vi "Check_Connections_between_Displ_in_Tracks-1.vi"(4 "error IN":errorcluster, 7 "[IN] Long Connected Tracks":T1(array[cluster])) -> (0 "error OUT":errorcluster, 3 "[OUT] Long Connected Tracks":T1(array[cluster]))   [LabVIEW 2013]
panel:
  out "Number of Unconnected Points":u8
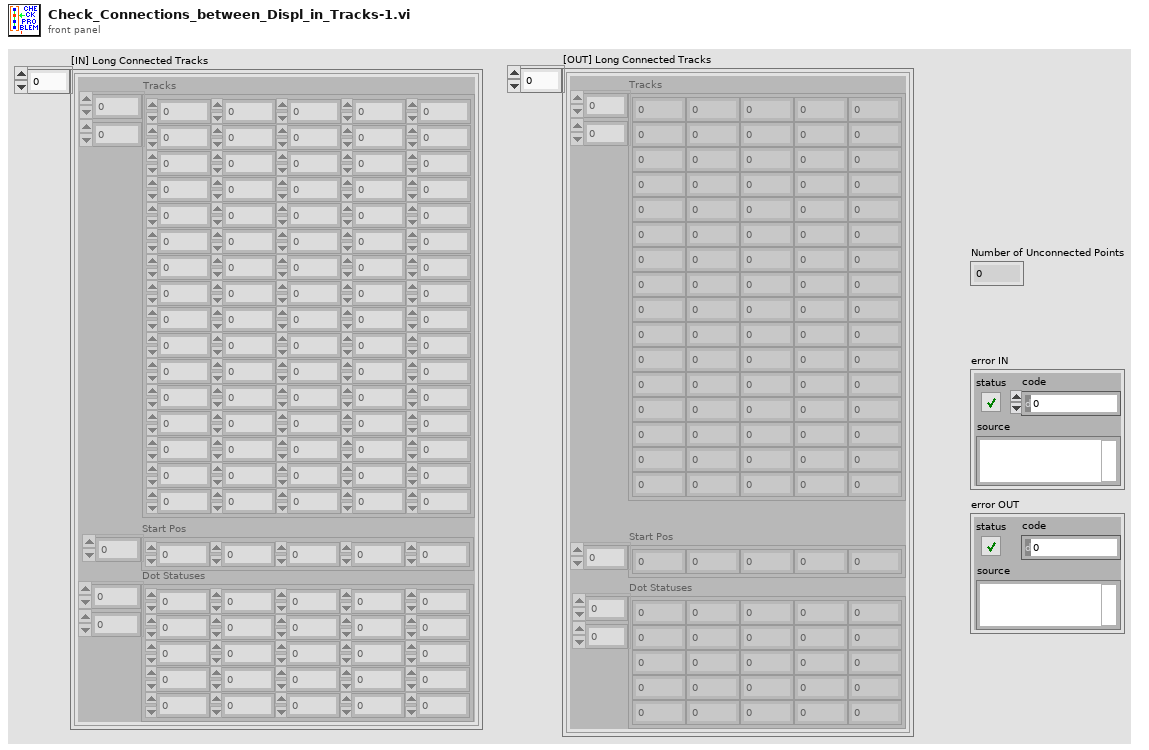
[diagram p1: front panel]
types:
  T1 = cluster{"Tracks":dbl[][], "Start Pos":i32[], "Dot Statuses":i16[][]}[]
  T2 = cluster{"Tracks":dbl[][], "Start Pos":i32[], "Dot Statuses":i16[][]}
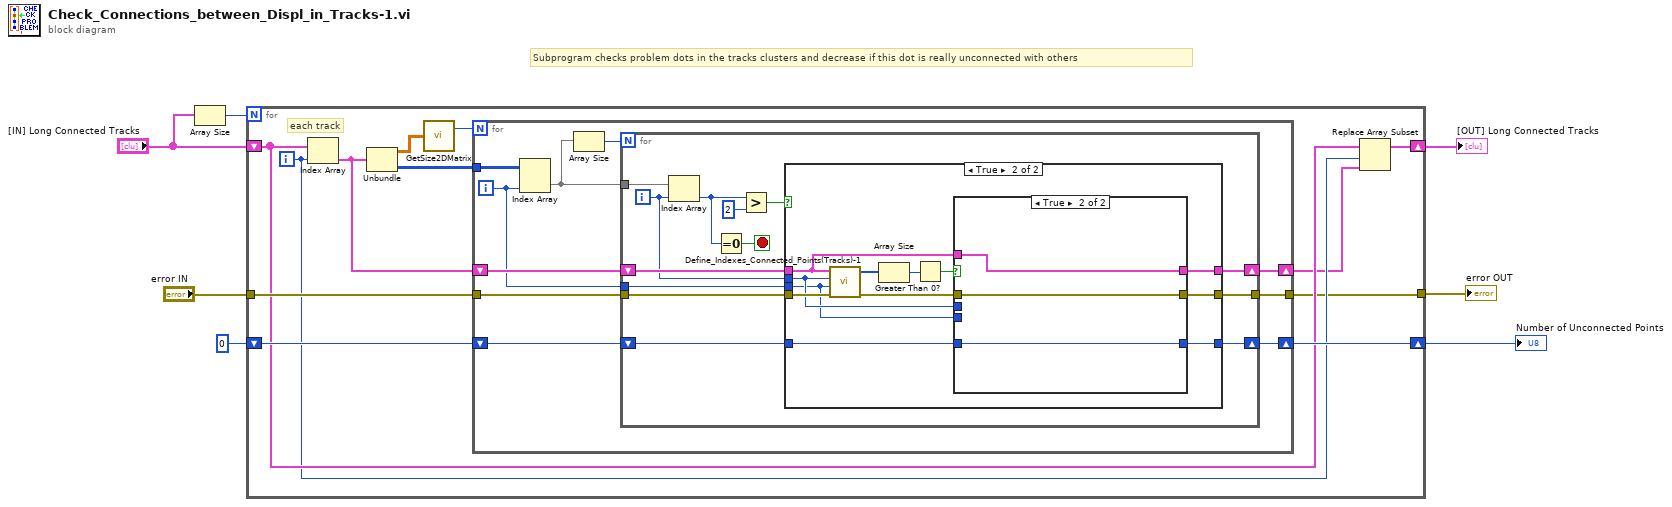
[diagram p0: block diagram]
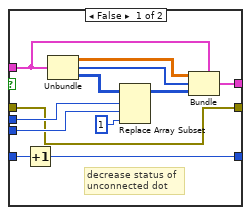
[diagram p3: hidden frame]
diagram:
  # "Subprogram checks problem dots in the tracks clusters and decrease if this dot is really unconnected with others"
  n1 = Array Size(array="[IN] Long Connected Tracks") -> (size(s)=w7:i32)
  n2 = for {
    N: w7 -> [_]
    shift-right: [w9] -> w2
    shift-left: "[IN] Long Connected Tracks" -> [w12]
    tunnel: "error IN" -> [w15]
    shift-right: [w13] -> w1
    shift-left: u8 0 -> [w14]
    tunnel: [w8] -> w3
    i -> [w11]
    # "each track"
    n3 = Index Array(array=w12, index=w11) -> (element=w16:T2)
    n4 = Unbundle(w16) -> ("Tracks"=w19:dbl[][], "Dot Statuses"=w17:i16[][])  [unwired: 1 out]
    n5 = call "GetSize2DMatrix.vi"("Array IN (2D)"=w19) -> ("# Cols"=w18:i32)  [unwired: 1 out]
    n6 = for {
      N: w18 -> [_]
      tunnel: w17 -> [w29]
      shift-right: [w23] -> w10
      shift-left: w16 -> [w26]
      tunnel: w15 -> [w24]
      shift-right: [w21] -> w13
      shift-left: w14 -> [w22]
      tunnel: [w20] -> w8
      i -> [w25]
      n7 = Index Array(array=w29, index (col)=w25) -> (element=w27:i16[])  [unwired: 1 in]
      n8 = Array Size(array=w27) -> (size(s)=w28:i32)
      n9 = for {
        N: w28 -> [_]
        tunnel: w27 -> [w42]
        shift-right: [w33] -> w23
        shift-left: w26 -> [w38]
        tunnel: w25 -> [w35]
        tunnel: w24 -> [w34]
        shift-right: [w31] -> w21
        shift-left: w22 -> [w32]
        tunnel: [w30] -> w20
        i -> [w36]
        stop <- w41 stop-if-true
        n10 = Index Array(array=w42, index=w36) -> (element=w37:i16)
        n11 = Equal To 0?(x=w37) -> (x = 0?=w41:bool)
        n12 = Greater?(x=w37, y=i16 2) -> (0:w39:bool)
        n13 = case shown="True" w39 {
          tunnel: w38 -> [w45 w53]
          tunnel: w36 -> [_ w49]
          tunnel: w35 -> [_ w48]
          tunnel: w34 -> [w44 w57]
          tunnel: [w45 w52] -> w33
          tunnel: w32 -> [w43 w51]
          tunnel: [w43 w50] -> w31
          tunnel: [w44 w46] -> w30
          frame False {
          }
          frame True {
            n14 = call "Define_Indexes_Connected_Points(Tracks)-1.vi"("error IN"=w57, "[IN] Index of track with\n(problem displacement)"=w48, "[IN]Index of problem\ndisplacement inside track"=w49, "[IN] Track group"=w53) -> ("error OUT"=w47:errorcluster, "[OUT] Index of connected\ntracks with problem dot"=w56:i32[])  [unwired: 1 out]
            n15 = Array Size(array=w56) -> (size(s)=w55:i32)
            n16 = Greater Than 0?(x=w55) -> (x > 0?=w54:bool)
            n17 = case shown="True" w54 {
              tunnel: w53 -> [w67 w72]
              tunnel: [w66 w72] -> w52
              tunnel: w51 -> [w69 w70]
              tunnel: [w68 w70] -> w50
              tunnel: w49 -> [w64 _]
              tunnel: w48 -> [w63 _]
              tunnel: w47 -> [w58 w71]
              tunnel: [w58 w71] -> w46
              frame False {
                # "decrease status of \nunconnected dot"
                n18 = Increment(x=w69) -> (x+1=w68:u8)
                n19 = Unbundle(w67) -> ("Tracks"=w62:dbl[][], "Start Pos"=w61:i32[], "Dot Statuses"=w65:i16[][])
                n20 = Replace Array Subset(array=w65, new element=i16 1 ("new element/subarray"), index (row)=w64, index (col)=w63) -> (w60:i16[][])
                n21 = Bundle(cluster=w67, "Tracks"=w62, "Start Pos"=w61, "Dot Statuses"=w60) -> (w66:T2)
              }
              frame True {
              }
            }
          }
        }
      }
    }
    n22 = Replace Array Subset(array=w12, new element=w10, index=w11) -> (w9:T1)
  }
  "error OUT" <- w3
  "[OUT] Long Connected Tracks" <- w2
  "Number of Unconnected Points" <- w1
